vi "Simple Network Streams - Host.vi"() -> ()   [LabVIEW 2023]
doc: "Demonstrates how to use network streams to pass data and commands between two running VIs. It displays waveform data that is received from the target VI and sends commands to update the frequency of the generated signal."
uses:
  support/Network Stream Command.ctl
  support/Network Stream Global Stop.vi
  <vilib>/ErrorRing/Error Ring.xnode
  <resource>/objmgr/ni.dex.rc
panel:
  in  "Read Speed":u16(ring)=1 items=["Fast (10 ms)", "Slow (20 ms)"]
  out "Read Backlog":i32
  in  "Frequency":dbl(knob)=10.1 scale=10.0..100.0
  in  "Stop":bool
  in  "Target IP Address":string="localhost"
  out "Acquired Data":waveform(dbl)[](graph)
  # "Overview: Demonstrates how to use Network Streams to pass data and commands between two running VIs.\nRequirements: Windows\nInstructions:\n1. Make sure Simple Network Streams - Target.vi is already running.\n2. Run this VI.\n3. Change the Frequency value and observe the change in data that results from sending the new frequency value to the Target VI.\n4. Change the Read Speed value in this VI, and the Write Speed value in the Target VI, and observe the resulting values of Read Backlog and Write Backlog.\n5. Click Stop to stop the VI."
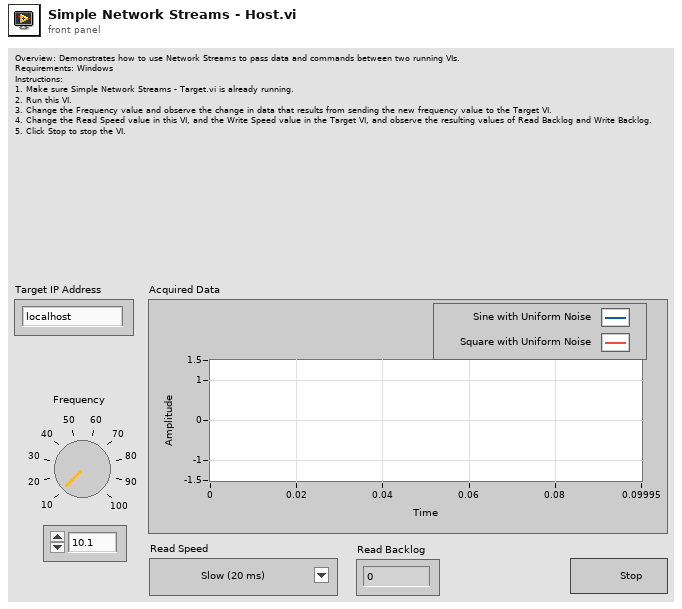
[diagram p1: front panel]
types:
  T1 = typedef "Network Stream Command.ctl" = cluster{"Message":string, "Message Data":variant}
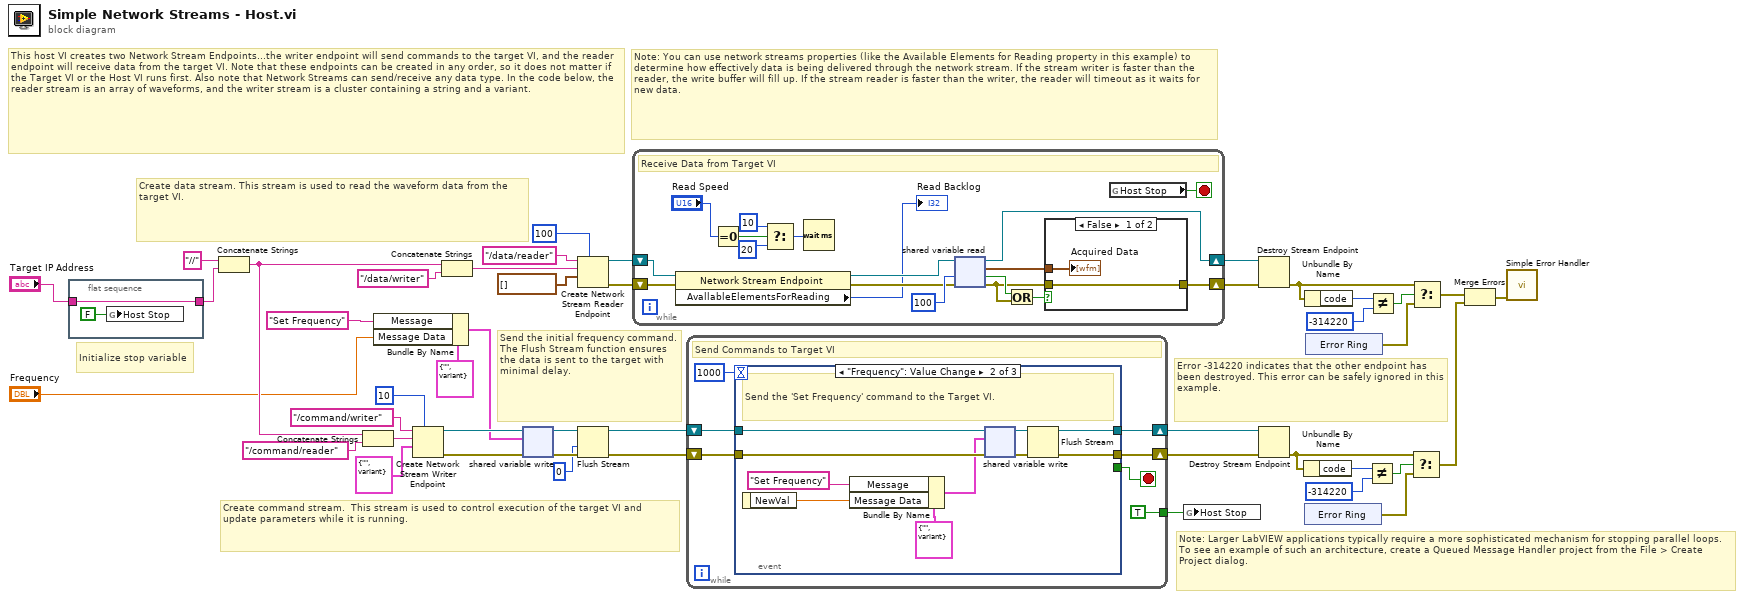
[diagram p0: block diagram]
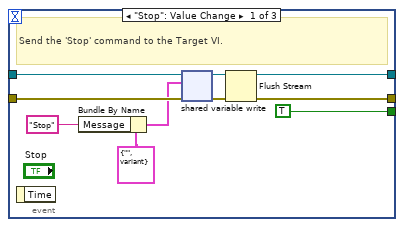
[diagram p3: hidden frame]
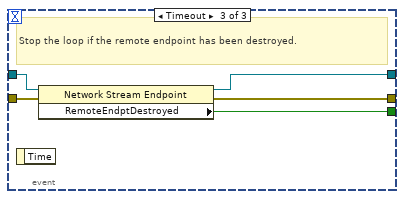
[diagram p4: hidden frame]
diagram:
  # "This host VI creates two Network Stream Endpoints...the writer endpoint will send commands to the target VI, and the reader endpoint will receive data from the target VI. Note that these endpoints can be created in any order, so it does not matter if the Target VI or the Host VI runs first. Also note that Network Streams can send/receive any data type. In the code below, the reader stream is an array of waveforms, and the writer stream is a cluster containing a string and a variant."
  # "Initialize stop variable"
  # "Note: Larger LabVIEW applications typically require a more sophisticated mechanism for stopping parallel loops. To see an example of such an architecture, create a Queued Message Handler project from the File > Create Project dialog."
  # "Error -314220 indicates that the other endpoint has been destroyed. This error can be safely ignored in this example."
  # "Note: You can use network streams properties (like the Available Elements for Reading property in this example) to determine how effectively data is being delivered through the network stream. If the stream writer is faster than the reader, the write buffer will fill up. If the stream reader is faster than the writer, the reader will timeout as it waits for new data."
  # "Create data stream. This stream is used to read the waveform data from the target VI."
  # "Create command stream.  This stream is used to control execution of the target VI and update parameters while it is running."
  # "Send the initial frequency command. The Flush Stream function ensures the data is sent to the target with minimal delay."
  n1 = flat-sequence {
    tunnel: "Target IP Address" -> [w47]
    tunnel: [w47] -> w1
    frame #0 {
      n2 = global write "Network Stream Global Stop.vi" "Host Stop"(FALSE ("Host Stop")) -> ()
    }
  }
  n3 = Concatenate Strings("//" ("reader url"), w1) -> (w35:string)
  n4 = Concatenate Strings(w35, "/command/reader" ("reader url")) -> (w36:string)
  n5 = Bundle By Name(cluster=T1 {"Message"="", "Message Data"=variant} ("Message Cluster"), "Message"="Set Frequency" ("Name"), "Message Data"="Frequency") -> (w19:T1)
  n6 = Create Network Stream Writer Endpoint(7:10 ("writer buffer size"), 9:T1 {"Message"="", "Message Data"=variant} ("Message Cluster"), 10:w36, 11:"/command/writer" ("writer name")) -> (0:w24:errorcluster, 3:w25:refnum<k21>)  [unwired: 3 in]
  n7 = Concatenate Strings(w35, "/data/writer" ("reader url")) -> (w37:string)
  n8 = shared-variable-write(w25, w24, w19) -> (w40:refnum<k21>, w30:errorcluster)  [unwired: 1 in, 1 out]
  n9 = Create Network Stream Reader Endpoint(7:100 ("reader buffer size"), 9:waveform(dbl)[] [], 10:w37, 11:"/data/reader" ("writer name")) -> (0:w43:errorcluster, 3:w42:refnum<k21>)  [unwired: 3 in]
  n10 = Flush Stream(8:w30, 9:0 ("timeout in ms (-1)"), 11:w40) -> (0:w29:errorcluster, 3:w31:refnum<k21>)  [unwired: 1 in, 1 out]
  n11 = while "Target->Host Data Reader" {
    shift-right: [w64] -> w23
    shift-left: w43 -> [w56]
    shift-right: [w61] -> w41
    shift-left: w42 -> [w58]
    stop <- w48 stop-if-true
    # "Receive Data from Target VI"
    n12 = property class="Network Stream Endpoint"(reference=w58, error in=w56) -> (reference out=w57:refnum<k21>, error out=w55:errorcluster, "AvallableElementsForReading"=→"Read Backlog":i32)
    n13 = Equal To 0?(x="Read Speed") -> (x = 0?=w52:bool)
    n14 = Select(t=u32 10 ("milliseconds to wait"), s=w52, f=u32 20 ("milliseconds to wait")) -> (s? t:f=w50:u32)
    n15 = Wait (ms)(milliseconds to wait=w50) -> ()  [unwired: 1 out]
    n16 = shared-variable-read(w57, w55, 100 ("timeout ms")) -> (w61:refnum<k21>, w60:errorcluster, w63:bool, w65:waveform(dbl)[])
    n17 = Or(x=w63, y=w60) -> (x .or. y?=w62:bool)
    n18 = case shown="False" w62 {
      tunnel: w65 -> [w66 _]
      tunnel: w60 -> [w67 w68]
      tunnel: [w67 w68] -> w64
      frame False {
        "Acquired Data" <- w66
      }
      frame True {
      }
    }
    n19 = global read "Network Stream Global Stop.vi" "Host Stop"() -> (w48:bool)
  }
  n20 = while "Host->Target Command Writer" {
    shift-right: [w72] -> w22
    shift-left: w29 -> [w74]
    shift-right: [w73] -> w27
    shift-left: w31 -> [w75]
    tunnel: [TRUE] -> w3
    stop <- w70 stop-if-true
    # "Send Commands to Target VI"
    n21 = event shown="[1] \"Frequency\": Value Change" {
      selector: _ -> [_ _ _]
      dyn-events: _ -> [_ _ _]
      timeout: 1000 -> [_ _ _]
      tunnel: w75 -> [w80 w94 w100]
      tunnel: w74 -> [w84 w93 w99]
      tunnel: [w81 w90 w98] -> w72
      tunnel: [w83 w92 w97] -> w73
      tunnel: [TRUE _ w96] -> w70
      event "Stop": Value Change {
        # "Send the 'Stop' command to the Target VI."
        n22 = event-data() -> ()  [unwired: 2 out]
        n23 = Bundle By Name(cluster=T1 {"Message"="", "Message Data"=variant} ("Message Cluster"), "Message"="Stop" ("Name")) -> (w78:T1)
        n24 = shared-variable-write(w80, w84, w78) -> (w85:refnum<k21>, w82:errorcluster)  [unwired: 1 in, 1 out]
        n25 = Flush Stream(8:w82, 11:w85) -> (0:w81:errorcluster, 3:w83:refnum<k21>)  [unwired: 2 in, 1 out]
      }
      event "Frequency": Value Change {
        # "Send the 'Set Frequency' command to the Target VI."
        n26 = event-data() -> ("NewVal"=w87:dbl)  [unwired: 1 out]
        n27 = Bundle By Name(cluster=T1 {"Message"="", "Message Data"=variant} ("Message Cluster"), "Message"="Set Frequency" ("Name"), "Message Data"=w87) -> (w86:T1)
        n28 = shared-variable-write(w94, w93, w86) -> (w95:refnum<k21>, w91:errorcluster)  [unwired: 1 in, 1 out]
        n29 = Flush Stream(8:w91, 11:w95) -> (0:w90:errorcluster, 3:w92:refnum<k21>)  [unwired: 2 in, 1 out]
      }
      event Timeout {
        # "Stop the loop if the remote endpoint has been destroyed."
        n30 = event-data() -> ()  [unwired: 2 out]
        n31 = property class="Network Stream Endpoint"(reference=w100, error in=w99) -> (reference out=w97:refnum<k21>, error out=w98:errorcluster, "RemoteEndptDestroyed"=w96:bool)
      }
    }
  }
  n32 = global write "Network Stream Global Stop.vi" "Host Stop"(w3) -> ()
  n33 = Destroy Stream Endpoint(8:w23, 11:w41) -> (0:w12:errorcluster)
  n34 = Destroy Stream Endpoint(8:w22, 11:w27) -> (0:w5:errorcluster)
  n35 = Unbundle By Name(w5) -> ("code"=w6:i32)
  n36 = Unbundle By Name(w12) -> ("code"=w15:i32)
  n37 = xnode "Error Ring"() -> ("error out"=w9:errorcluster)
  n38 = xnode "Error Ring"() -> ("error out"=w11:errorcluster)
  n39 = Not Equal?(x=w6, y=-314220) -> (x != y?=w8:bool)
  n40 = Not Equal?(x=w15, y=-314220) -> (x != y?=w13:bool)
  n41 = Select(t=w5, s=w8, f=w9) -> (s? t:f=w4:errorcluster)
  n42 = Select(t=w12, s=w13, f=w11) -> (s? t:f=w10:errorcluster)
  n43 = Merge Errors(w10, w4) -> (w26:errorcluster)
  n44 = call <vilib>:"Simple Error Handler.vi"("error in (no error)"=w26) -> ()  [unwired: 4 in, 5 out]
